vi "Handle Error.vi"(8 "error in (no error)":errorcluster, 11 "CO2 Actor in":refnum<class "CO2 Actor.lvclass">) -> (0 "error out":errorcluster, 2 "stop actor?":bool=TRUE, 3 "CO2 Actor out":refnum<class "CO2 Actor.lvclass">)   [LabVIEW 2015, in "cRIO-Carbondioxide.lvlib" / "CO2-Actor.lvlib" / "CO2 Actor.lvclass"]
doc: "(<B>Filename</B>: Actor Framework.lvlib:Actor.lvclass:Handle Error.vi)\n\nDefines how the actor handles an error that occurred while processing a message.\n\nBy default, this method does nothing except stop the actor. This method also treats error code 43 (coming from <B>error in</B>) as a sign that the actor shut down normally. In this situation, the Handle Error method does not return the error on <B>error out</B>, meaning the actor's caller will not receive it. All other error codes will be returned on <B>error out</B>.\n\nA descendant class may override this method to change this behavior."
uses:
  CO2 Actor.lvclass
  <vilib>/ActorFramework/Actor/Actor.lvclass
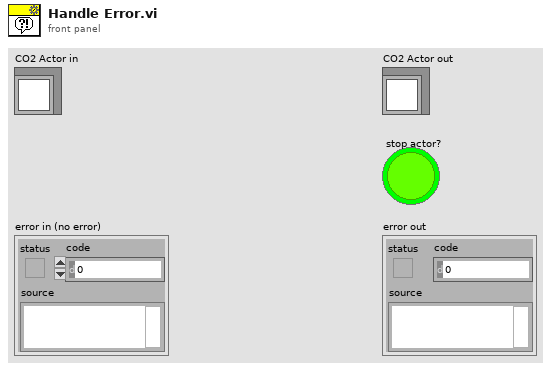
[diagram p1: front panel]
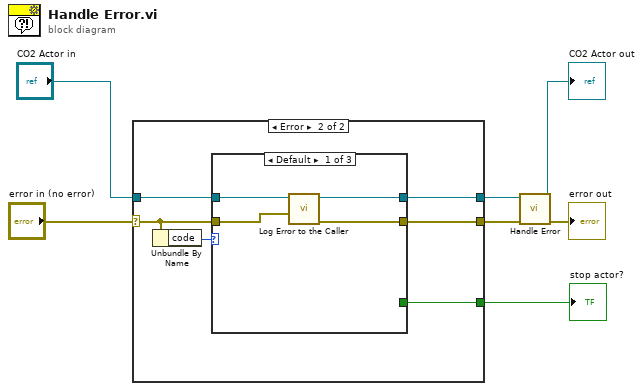
[diagram p0: block diagram]
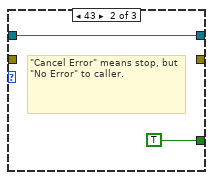
[diagram p3: hidden frame]
diagram:
  n1 = case shown="Error" "error in (no error)" {
    selector: "error in (no error)" -> [w9 w12]
    tunnel: [w9 w15] -> w5
    tunnel: [_ w13] -> w4
    tunnel: "CO2 Actor in" -> [w8 w11]
    tunnel: [w8 w10] -> w1
    frame No Error {
    }
    frame Error {
      n2 = Unbundle By Name(w12) -> ("code"=w14:i32)
      n3 = case shown="Default" w14 {
        tunnel: w12 -> [w17 _ _]
        tunnel: [w16 _ _] -> w15
        tunnel: [_ TRUE ("stop actor?") _] -> w13
        tunnel: w11 -> [w19 w20 w22]
        tunnel: [w18 w20 w22] -> w10
        frame Default {
          n4 = call-dynamic "Log Error to the Caller.vi"("Error to log"=w17, "CO2 Actor in"=w19) -> ("error out"=w16:errorcluster, "CO2 Actor out"=w18:refnum<class "CO2 Actor.lvclass">)  [unwired: 8 in]
        }
        frame 43 {
          # "\"Cancel Error\" means stop, but \"No Error\" to caller."
        }
        frame 1448 {
          # "Bad type cast. Happens when a message is not ment for the Actor."
        }
      }
    }
  }
  "stop actor?" <- w4
  n5 = call-parent "Handle Error.vi"("error in (no error)"=w5, "Actor in"=w1) -> ("error out"=→"error out":errorcluster, "Actor out"=→"CO2 Actor out":refnum<class "CO2 Actor.lvclass">)  [unwired: 7 in, 1 out]
